vi "(SubVI)Run Script.vi"(7 "GUI Log Obj":refnum<class "GUI Log Class.lvclass">, 8 "error in (no error)":errorcluster caption="에러 입력(에러 없음)", 10 "Script Content":string, 11 "Script File":path) -> (0 "error out":errorcluster caption="에러 출력")   [LabVIEW 2020]
uses:
  Libraries/GUI Log Class/GUI Log Class/GUI Log Class.lvclass
  Libraries/Script Line Class/Script Line/Script Line.lvclass
panel:
  in  "Stop":bool
  out "Status":string
  out "Progress Bar":i32(slide)=-1 scale=0.0..2.0
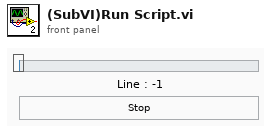
[diagram p1: front panel]
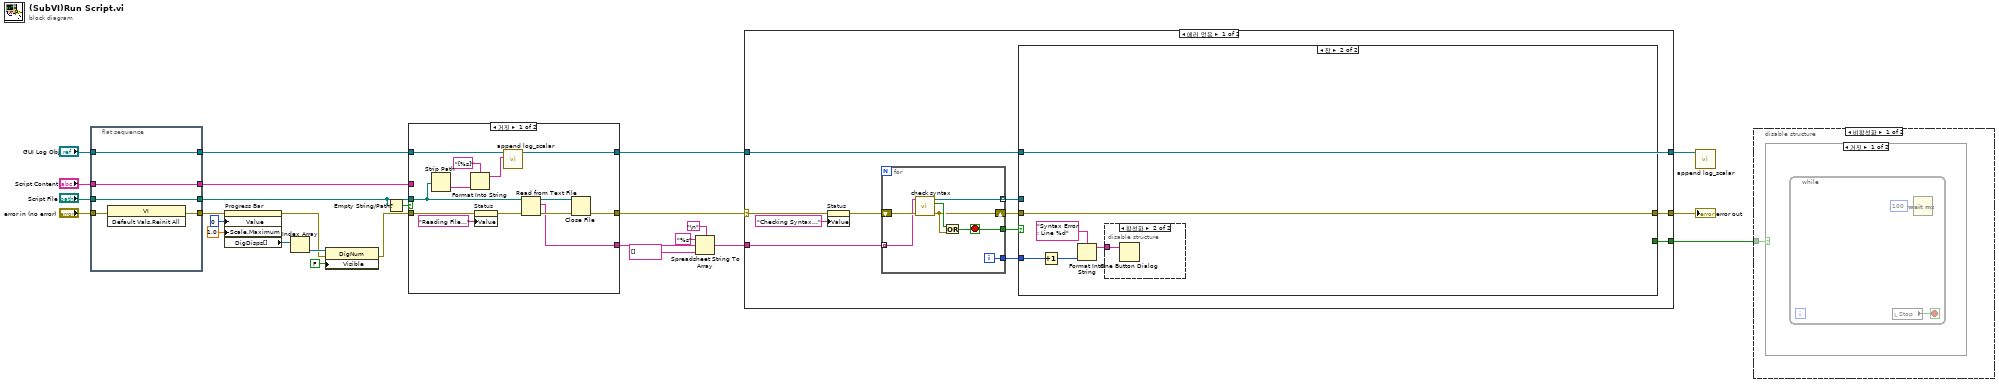
[diagram p0: block diagram]
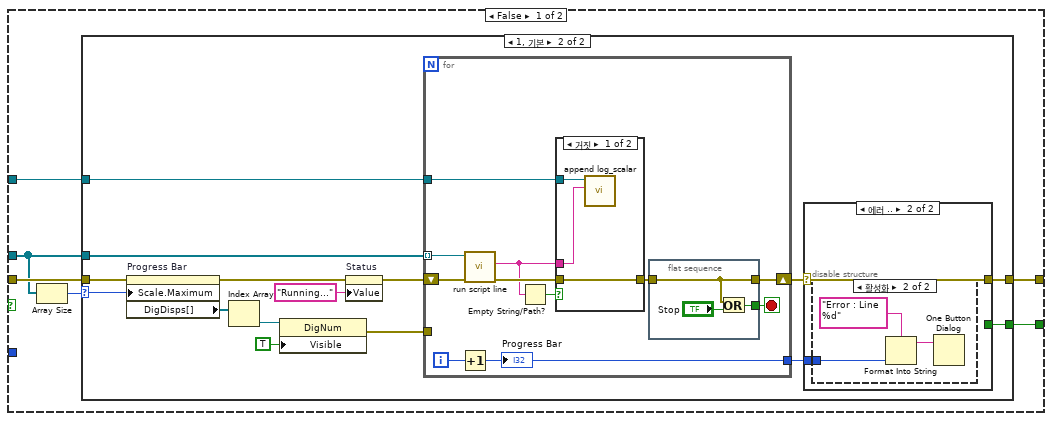
[diagram p5: hidden frame]
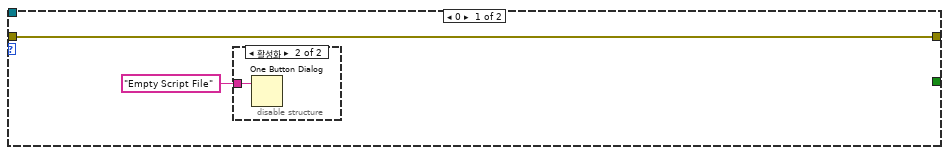
[diagram p6: hidden frame]
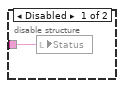
[diagram p7: hidden frame]
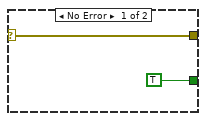
[diagram p8: hidden frame]
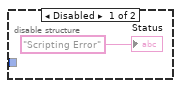
[diagram p9: hidden frame]
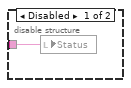
[diagram p11: hidden frame]
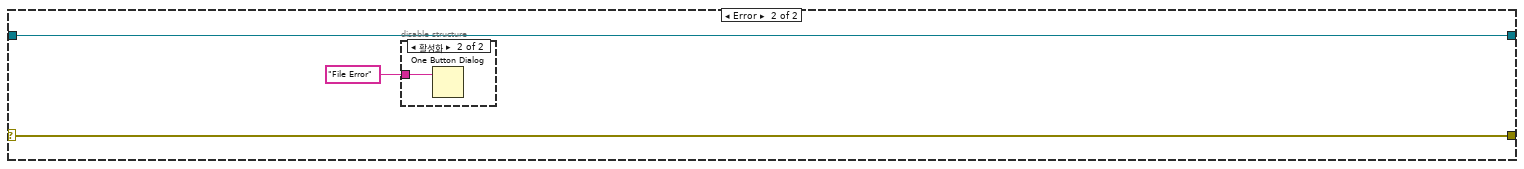
[diagram p12: hidden frame]
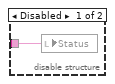
[diagram p13: hidden frame]
diagram:
  n1 = flat-sequence {
    tunnel: "error in (no error)" -> [w31]
    tunnel: [w30] -> w22
    tunnel: "Script File" -> [w28]
    tunnel: "GUI Log Obj" -> [w29]
    tunnel: [w29] -> w3
    tunnel: [w28] -> w11
    tunnel: [w27] -> w9
    tunnel: "Script Content" -> [w27]
    frame #0 {
      n2 = invoke class="VI" method="Default Vals.Reinit All"(error in=w31) -> (error out=w30:errorcluster)  [unwired: 2 in, 2 out]
    }
  }
  n3 = property on="Progress Bar" class="Slide (엄격한)"(error in=w22, "Value"=0 ("Progress Bar"), "Scale.Maximum"=1.0 ("스케일.범위:최대값")) -> (error out=w18:errorcluster, "DigDisps[]"=w21:refnum<vi>[])  [unwired: 1 in, 1 out]
  n4 = Index Array(array=w21) -> (element=w20:refnum<vi>)  [unwired: 1 in]
  n5 = property class="DigNum"(reference=w20, error in=w18, "Visible"=FALSE ("보이기")) -> (error out=w17:errorcluster)  [unwired: 1 out]
  n6 = Empty String/Path?(string/path=w11) -> (empty?=w10:bool)
  n7 = case shown="거짓" w10 {
    tunnel: [w40 w47] -> w24
    tunnel: w17 -> [w39 w47]
    tunnel: w11 -> [w35 _]
    tunnel: w9 -> [_ w46]
    tunnel: [w38 w46] -> w5
    tunnel: w3 -> [w37 w45]
    tunnel: [w36 w45] -> w2
    frame False {
      n8 = Strip Path(path=w35) -> (name=w33:string)  [unwired: 1 out]
      n9 = Format Into String(format string="[%s]" ("포맷 문자열"), w33) -> (resulting string=w32:string)  [unwired: 2 in, 1 out]
      n10 = property on="Status" class="Str"(error in=w39, "Value"="Reading File..." ("Status")) -> (error out=w41:errorcluster)  [unwired: 1 in, 1 out]
      n11 = call-dynamic "append log_scalar.vi"("log to append"=w32, "GUI Log Class 입력"=w37) -> ("GUI Log Class 출력"=w36:refnum<class "GUI Log Class.lvclass">)  [unwired: 8 in, 1 out]
      n12 = Read from Text File(file (use dialog)=w35, error in=w41) -> (refnum out=w44:refnum<file>, text=w38:string, error out=w43:errorcluster)  [unwired: 2 in, 1 out]
      n13 = Close File(refnum=w44, error in=w43) -> (error out=w40:errorcluster)  [unwired: 1 out]
    }
    frame True {
    }
  }
  n14 = Spreadsheet String To Array(delimiter (Tab)="\n", format string="%s" ("포맷 문자열"), spreadsheet string=w5, array type (2D Dbl)=string[] []) -> (array=w4:string[])
  n15 = case shown="에러 없음" w24 {
    selector: w24 -> [w52 w126]
    tunnel: w4 -> [w56 _]
    tunnel: [w54 w126] -> w16
    tunnel: w2 -> [w48 w124]
    tunnel: [w49 _] -> w15
    tunnel: [w48 w124] -> w1
    frame No Error {
      n16 = property on="Status" class="Str"(error in=w52, "Value"="Checking Syntax..." ("Status")) -> (error out=w51:errorcluster)  [unwired: 1 in, 1 out]
      n17 = for {
        tunnel: [w65] -> w58 mode=indexing
        shift-right: [w61] -> w57
        shift-left: w51 -> [w64]
        tunnel: w56 -> [w63] mode=indexing
        tunnel: [w60] -> w55
        tunnel: [w59] -> w50
        i -> [w59]
        stop <- w60 stop-if-true
        n18 = call "check syntax.vi"("error in (no error)"=w64, "script"=w63) -> ("error out"=w61:errorcluster, "error"=w62:bool, "Script Line 출력"=w65:refnum<class "Script Line.lvclass">)  [unwired: 3 in, 4 out]
        n19 = Or(x=w62, y=w61) -> (x .or. y?=w60:bool)
      }
      n20 = case shown="참" w55 {
        tunnel: w58 -> [w68 _]
        tunnel: w57 -> [w69 w121]
        tunnel: [w71 w121] -> w54
        tunnel: w48 -> [w70 _]
        tunnel: w50 -> [_ w118]
        tunnel: [w66 _] -> w49
        frame False {
          n21 = Array Size(array=w68) -> (size(s)=w67:i32)
          n22 = case shown="1, 기본" w67 {
            selector: w67 -> [_ w87]
            tunnel: [w73 w82] -> w71
            tunnel: w70 -> [_ w90]
            tunnel: w69 -> [w73 w89]
            tunnel: w68 -> [_ w88]
            tunnel: [_ w76] -> w66
            frame 0 {
              n23 = disable-structure shown="활성화" {
                disable-tunnel: "Empty Script File" ("Status") -> [w74 w75]
                frame Disabled {
                  n24 = local write "Status"(w74) -> ()
                }
                frame Enabled {
                  n25 = One Button Dialog(message=w75) -> ()  [unwired: 1 in, 1 out]
                }
              }
            }
            frame 1, Default {
              n26 = property on="Progress Bar" class="Slide (엄격한)"(error in=w89, "Scale.Maximum"=w87) -> (error out=w86:errorcluster, "DigDisps[]"=w80:refnum<vi>[])  [unwired: 1 in, 1 out]
              n27 = Index Array(array=w80) -> (element=w79:refnum<vi>)  [unwired: 1 in]
              n28 = property class="DigNum"(reference=w79, "Visible"=TRUE ("보이기")) -> (error out=w77:errorcluster)  [unwired: 1 in, 1 out]
              n29 = property on="Status" class="Str"(error in=w86, "Value"="Running..." ("Status")) -> (error out=w84:errorcluster)  [unwired: 1 in, 1 out]
              n30 = for {
                tunnel: w88 -> [w109] mode=indexing
                shift-right: [w99] -> w83
                shift-left: w84 -> [w108]
                tunnel: w90 -> [w107]
                tunnel: [w101] -> w81
                tunnel: w77 -> [_]
                i -> [w102]
                stop <- w106 stop-if-true
                n31 = Increment(x=w102) -> (x+1=w101:i32)
                "Progress Bar" <- w101
                n32 = call-dynamic "run script line.vi"("error in (no error)"=w108, "Script Line 입력"=w109) -> ("error out"=w104:errorcluster, "log"=w103:string)  [unwired: 7 in, 1 out]
                n33 = Empty String/Path?(string/path=w103) -> (empty?=w100:bool)
                n34 = case shown="거짓" w100 {
                  tunnel: w104 -> [w113 w116]
                  tunnel: [w113 w116] -> w105
                  tunnel: w107 -> [w115 _]
                  tunnel: w103 -> [w114 _]
                  frame False {
                    n35 = call-dynamic "append log_scalar.vi"("log to append"=w114, "GUI Log Class 입력"=w115) -> ()  [unwired: 8 in, 2 out]
                  }
                  frame True {
                  }
                }
                n36 = flat-sequence {
                  tunnel: [w112] -> w106
                  tunnel: w105 -> [w110]
                  tunnel: [w110] -> w99
                  frame #0 {
                    n37 = Or(x=w110, y="Stop") -> (x .or. y?=w112:bool)
                  }
                }
              }
              n38 = case shown="에러 .." w83 {
                selector: w83 -> [w92 w94]
                tunnel: [w92 w94] -> w82
                tunnel: w81 -> [_ w93]
                tunnel: [TRUE _] -> w76
                frame No Error {
                }
                frame Error {
                  n39 = disable-structure shown="활성화" {
                    disable-tunnel: w93 -> [_ w97]
                    frame Disabled {
                      "Status" <- "Scripting Error" ("Status")
                    }
                    frame Enabled {
                      n40 = Format Into String(format string="Error : Line %d" ("포맷 문자열"), w97) -> (resulting string=w96:string)  [unwired: 2 in, 1 out]
                      n41 = One Button Dialog(message=w96) -> ()  [unwired: 1 in, 1 out]
                    }
                  }
                }
              }
            }
          }
        }
        frame True {
          n42 = Increment(x=w118) -> (x+1=w117:i32)
          n43 = Format Into String(format string="Syntax Error : Line %d" ("포맷 문자열"), w117) -> (resulting string=w120:string)  [unwired: 2 in, 1 out]
          n44 = disable-structure shown="활성화" {
            disable-tunnel: w120 -> [w122 w123]
            frame Disabled {
              n45 = local write "Status"(w122) -> ()
            }
            frame Enabled {
              n46 = One Button Dialog(message=w123) -> ()  [unwired: 1 in, 1 out]
            }
          }
        }
      }
    }
    frame Error {
      n47 = disable-structure shown="활성화" {
        disable-tunnel: "File Error" ("Status") -> [w127 w128]
        frame Disabled {
          n48 = local write "Status"(w127) -> ()
        }
        frame Enabled {
          n49 = One Button Dialog(message=w128) -> ()  [unwired: 1 in, 1 out]
        }
      }
    }
  }
  "error out" <- w16
  n50 = call-dynamic "append log_scalar.vi"("GUI Log Class 입력"=w1) -> ()  [unwired: 9 in, 2 out]
  n51 = disable-structure shown="비활성화" {
    disable-tunnel: w15 -> [w129 _]
    frame Disabled {
      n52 = case shown="거짓" w129 {
        frame False {
          n53 = while {
            stop <- w131 stop-if-true
            n54 = local read "Stop"() -> (w131:bool)
            n55 = Wait (ms)(milliseconds to wait=u32 100 ("대기 시간 (ms)")) -> ()  [unwired: 1 out]
          }
        }
        frame True {
        }
      }
    }
    frame Enabled {
    }
  }
